vi "LEBITplc.CreateDBArray.vi"(0 "connection in":refnum<k7>, 2 "query results":string[][](array[string]), 5 "error in":errorcluster, 8 "Associated Panels":string[](array[string])=["Buncher", "TestIonSource", "Penning", "BuntoPenning", "PenningEject", "Mcp&PhosVol", "GasCell", "IonGuide", "N4toBob1", "Bob1toBun", "DeceltoBun", "LAS"]) -> (14 "connection out":refnum<k7>, 15 "InfoArray":string[][](array[string]), 18 "DBArray":string[][](array[string]), 19 "error out":errorcluster)   [LabVIEW 2014, in "LEBITplc.lvlib"]
uses:
  LEBITplc.lvlib
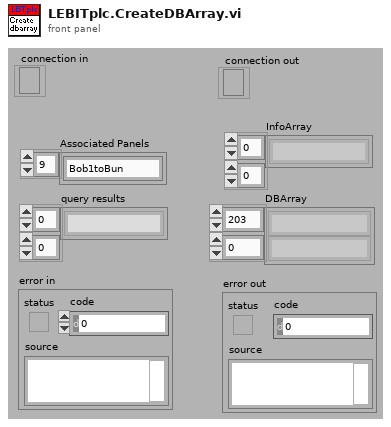
[diagram p1: front panel]
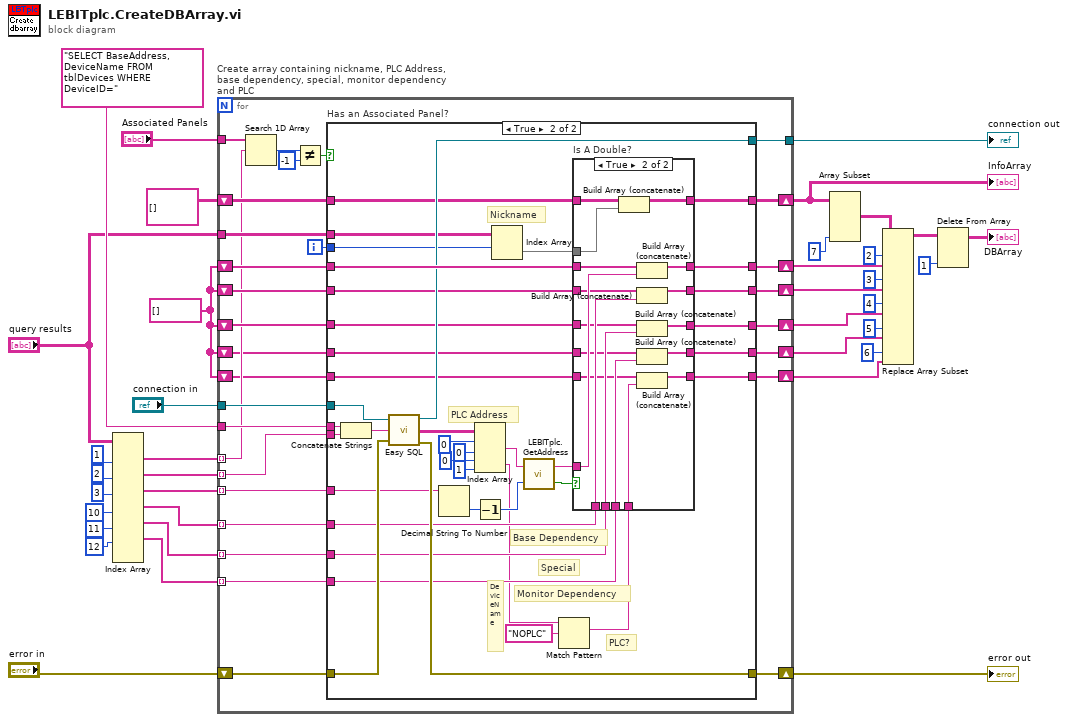
[diagram p0: block diagram]
diagram:
  w3 = string[] []
  n1 = Index Array(array="query results", index (col) #1=1 ("disabled index (col)"), index (col) #2=2 ("disabled index (col)"), index (col) #3=3 ("index (col)"), index (col) #4=10 ("index (col)"), index (col) #5=11 ("index (col)"), index (col) #6=12 ("index (col)")) -> (element #1=w8:string[], element #2=w26:string[], element #3=w29:string[], element #4=w22:string[], element #5=w20:string[], element #6=w4:string[])  [unwired: 8 in, 1 out]
  n2 = for "Create array containing nickname, PLC Address, base dependency, special, monitor dependency and PLC" {
    tunnel: w26 -> [w38] mode=indexing
    tunnel: "connection in" -> [w66]
    tunnel: w29 -> [w63] mode=indexing
    shift-right: [w62] -> w32
    shift-left: "error in" -> [w65]
    tunnel: "SELECT BaseAddress, DeviceName FROM tblDevices WHERE DeviceID=" -> [w64]
    shift-right: [w60] -> w35
    shift-left: w3 -> [w61]
    tunnel: w22 -> [w58] mode=indexing
    tunnel: w20 -> [w57] mode=indexing
    tunnel: [w59] -> w18
    shift-right: [w56] -> w16
    shift-left: w3 -> [w55]
    shift-right: [w54] -> w15
    shift-left: w3 -> [w53]
    tunnel: "query results" -> [w52]
    shift-right: [w49] -> w13
    shift-left: string[][] [] -> [w50]
    tunnel: "Associated Panels" -> [w48]
    tunnel: w8 -> [w47] mode=indexing
    shift-right: [w42] -> w6
    shift-left: w3 -> [w43]
    tunnel: w4 -> [w41] mode=indexing
    shift-right: [w39] -> w1
    shift-left: w3 -> [w40]
    i -> [w51]
    n3 = Search 1D Array(1D array=w48, element=w47) -> (index of element=w46:i32)  [unwired: 1 in]
    n4 = Not Equal?(x=w46, y=-1) -> (x != y?=w44:bool)
    n5 = case "Has an Associated Panel?" shown="True" w44 {
      tunnel: w66 -> [w74 w113]
      tunnel: w65 -> [w69 w112]
      tunnel: w64 -> [_ w111]
      tunnel: w38 -> [_ w110]
      tunnel: w63 -> [_ w80]
      tunnel: [w69 w107] -> w62
      tunnel: w61 -> [w72 w106]
      tunnel: [w72 w105] -> w60
      tunnel: [w74 w97] -> w59
      tunnel: w58 -> [_ w96]
      tunnel: w57 -> [_ w95]
      tunnel: [w71 w94] -> w56
      tunnel: w55 -> [w71 w93]
      tunnel: [w70 w92] -> w54
      tunnel: w53 -> [w70 w91]
      tunnel: w52 -> [_ w90]
      tunnel: w51 -> [_ w86]
      tunnel: w50 -> [w73 w89]
      tunnel: [w73 w88] -> w49
      tunnel: [w68 w85] -> w42
      tunnel: w43 -> [w68 w84]
      tunnel: w41 -> [_ w83]
      tunnel: w40 -> [w67 w82]
      tunnel: [w67 w81] -> w39
      frame False {
      }
      frame True {
        # "PLC?"
        # "DeviceName"
        # "Monitor Dependency"
        # "Nickname"
        # "Special"
        # "Base Dependency"
        # "PLC Address"
        n6 = Concatenate Strings(w111, w110) -> (w109:string)
        n7 = call <vilib>:"Easy SQL.vi"("connection"=w113, "SQL statement"=w109, "error in (no error)"=w112) -> ("connection"=w97:refnum<k7>, "error out"=w107:errorcluster, "query results"=w108:string[][])  [unwired: 2 out]
        n8 = Decimal String To Number(string=w80) -> (number=w103:i32)  [unwired: 2 in, 1 out]
        n9 = Index Array(array=w108, index (row) #1=0 ("index (row)"), index (col) #1=0 ("disabled index (col)"), index (row) #2=0 ("index (row)"), index (col) #2=1 ("disabled index (col)")) -> (element #1=w100:string, element #2=w75:string)
        n10 = Decrement(x=w103) -> (x-1=w101:i32)
        n11 = Index Array(array=w90, index (row)=w86) -> (element=w87:string[])  [unwired: 1 in]
        n12 = call "LEBITplc.GetAddress.vi"("channel# (dec)"=w101, "base Actual addr. (oct)"=w100) -> ("is a double?"=w98:bool, "act. addr. (oct)"=w99:string)
        n13 = Match Pattern(string=w75, regular expression="NOPLC") -> (match substring=w78:string)  [unwired: 1 in, 3 out]
        n14 = case "Is A Double?" shown="True" w98 {
          tunnel: w106 -> [w119 w137]
          tunnel: [w119 w136] -> w105
          tunnel: w99 -> [_ w135]
          tunnel: w96 -> [_ w134]
          tunnel: w95 -> [_ w133]
          tunnel: [w118 w132] -> w94
          tunnel: w93 -> [w118 w130]
          tunnel: [w117 w131] -> w92
          tunnel: w91 -> [w117 w129]
          tunnel: w89 -> [w116 w128]
          tunnel: [w116 w127] -> w88
          tunnel: w87 -> [_ w126]
          tunnel: [w115 w125] -> w85
          tunnel: w84 -> [w115 w124]
          tunnel: w83 -> [_ w123]
          tunnel: w82 -> [w114 w122]
          tunnel: [w114 w121] -> w81
          tunnel: w78 -> [_ w120]
          frame False {
          }
          frame True {
            n15 = Build Array (concatenate)(w128, w126) -> (w127:string[][])
            n16 = Build Array (concatenate)(w137, w135) -> (w136:string[])
            n17 = Build Array (concatenate)(w130, w134) -> (w132:string[])
            n18 = Build Array (concatenate)(w129, w133) -> (w131:string[])
            n19 = Build Array (concatenate)(w124, w123) -> (w125:string[])
            n20 = Build Array (concatenate)(w122, w120) -> (w121:string[])
          }
        }
      }
    }
  }
  "error out" <- w32
  "connection out" <- w18
  "InfoArray" <- w13
  n21 = Array Subset(array=w13, length (col)=7 ("length")) -> (w12:string[][])  [unwired: 3 in]
  n22 = Replace Array Subset(array=w12, new element #1=w35, index (col) #1=2 ("disabled index (col)"), new element #2=w16, index (col) #2=3 ("index (col)"), new element #3=w15, index (col) #3=4 ("index (col)"), new element #4=w6, index (col) #4=5 ("index (col)"), new element #5=w1, index (col) #5=6 ("index (col)")) -> (w36:string[][])  [unwired: 5 in]
  n23 = Delete From Array(array=w36, index (col)=1 ("disabled index (col)")) -> (array with subset deleted=→"DBArray":string[][])  [unwired: 2 in, 1 out]
